vi "CONEX-CC Virtual Front Panel_v2.vi"(6 "+":bool, 7 "-":bool, 8 "Set velocity":bool, 9 "Action":bool) -> ()   [LabVIEW 2016]
doc: "CONEX - CC Virtual Front Panel:\n\nThis is a sample of an application that can be built with the LabVIEW drivers.\n\nPress HOME / ENABLE in top left of panel to put stage in Ready state for motion."
uses:
  <vilib>/Platform/TimedLoop/XDataNode/timing_clust.ctl
  <vilib>/Platform/TimedLoop/XDataNode/nitl_modes.ctl
  <vilib>/Platform/TimedLoop/XDataNode/wakeup.ctl
  <vilib>/Platform/TimedLoop/XDataNode/XDataNode.xnode
  <vilib>/Platform/TimedLoop/XDataNode/XDNodeRunTimeDep.lvlib
panel:
  out "Title":string
  out "counter":i32
  in  "Set Max":bool
  in  "Set Min":bool
  in  "Max":dbl
  in  "Min":dbl
  out "Stop cycle":bool=TRUE
  out "Title 2":string
  in  "Cycle":bool
  in  "# Loops":i32=5
  in  "Go2":bool
  in  "Go1":bool
  in  "Abs. Move 2":dbl=1.0
  in  "Abs. Move 1":dbl
  in  "Step":dbl
  out "Position History":dbl(graph)=1.5
  out "Stop polling":bool=TRUE
  out "Controller state description":string="STATUS"
  out "Velocity MAX":dbl=0.4
  out "Controller state":string="33"
  out "Positioner error":string="0000"
  in  "Velocity:":dbl
  in  "Exit":bool=TRUE
  out "Target position":dbl
  in  "Position glissière":cluster{dbl, dbl}(slide) scale=0.0..25.0
  in  "Exit":bool
  out "Current position":dbl
  # "unit/s"
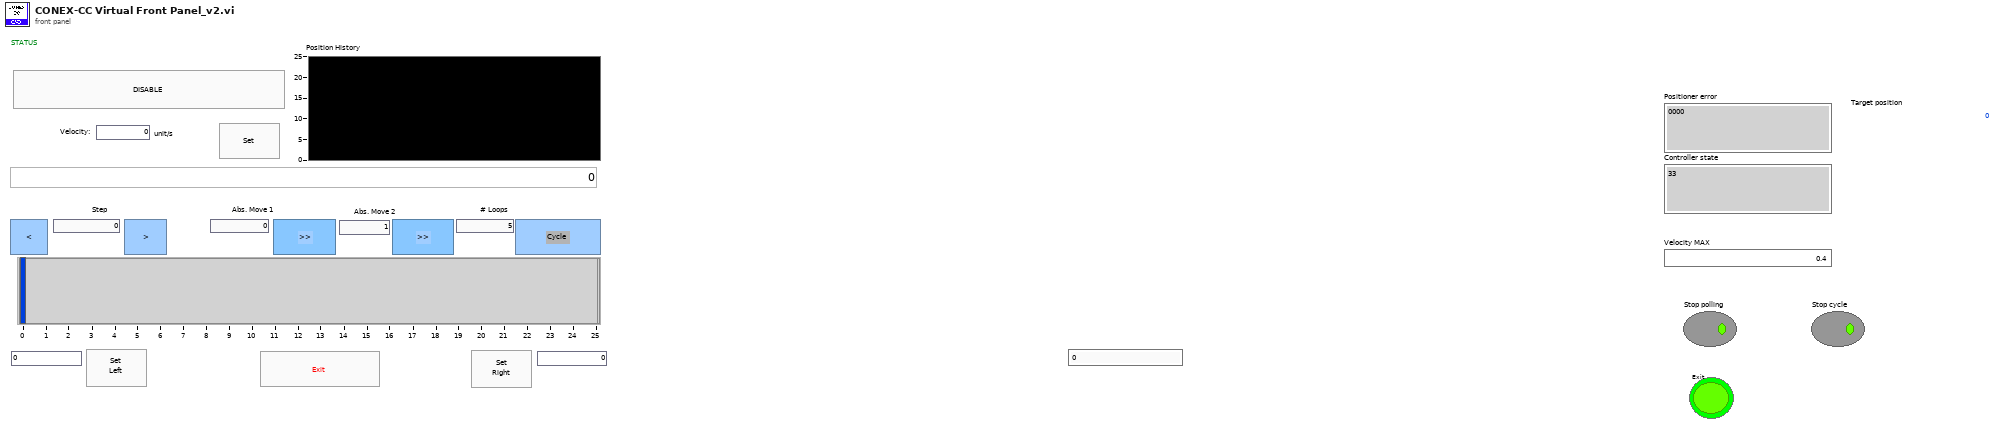
[diagram p1: front panel]
types:
  T1 = typedef "XDNodeRunTimeDep.lvlib/timing_clust.ctl" = cluster{"Expected End [f-1]":u64, "Actual End [f-1]":u64, "Finished Late? [f-1]":bool, "Expected End [i-1]":u64, "Actual End [i-1]":u64, "Finished Late? [i-1]":bool, "Expected Start [i]":u64, "Actual Start [i]":u64, "Expected Start [f]":u64, "Actual Start [f]":u64, "Source Name":string, "Structure Name":string, "Period":i64, "Deadline":i64, "Offset":i64, "Start":i64, "Priority":i32, "Timeout":i32, "Mode":T2, "Wakeup Reason":T3, "Error":errorcluster, "Source Type":string, "Secondary Source Type":string, "Global End Time":u64, "Global Start Time":u64, "Frame Duration":u64, "Iteration Duration":u64, "Assigned CPU":i32, "I/O Scan Engine Mode":u32}
  T2 = typedef "XDNodeRunTimeDep.lvlib/nitl_modes.ctl" = enum32{"No Change", "Process missed periods, maintain original phase", "Discard missed periods, maintain original phase", "Process missed periods, ignore original phase", "Discard missed periods, ignore original phase"}
  T3 = typedef "XDNodeRunTimeDep.lvlib/wakeup.ctl" = enum32{"Normal", "Aborted", "Asynchronous wakeup", "Timing source error", "Timed loop error", "Timeout"}
  T4 = cluster{"VISA resource name":refnum<visa-resource-name>, "Device name":string, "Controller address":i32, "error":errorcluster}
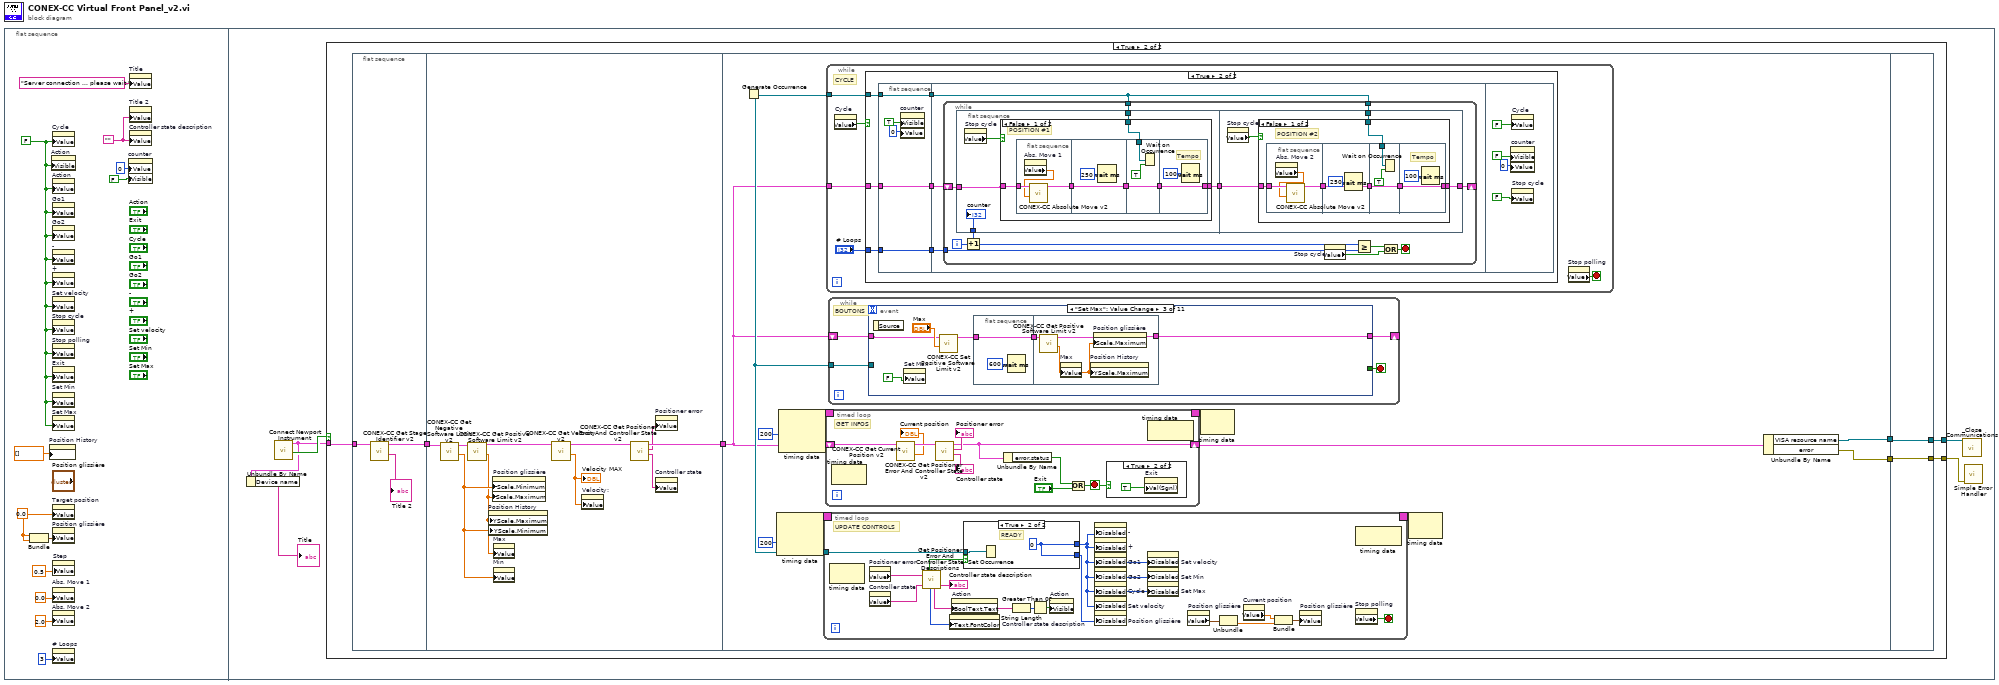
[diagram p0: block diagram]
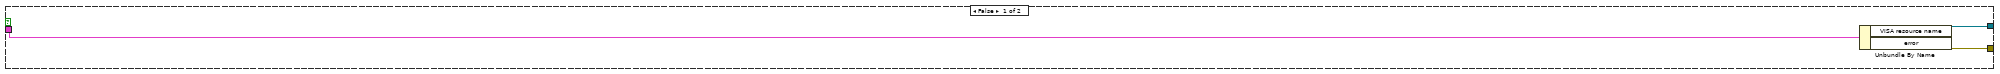
[diagram p2: hidden frame]
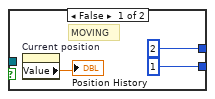
[diagram p6: hidden frame]
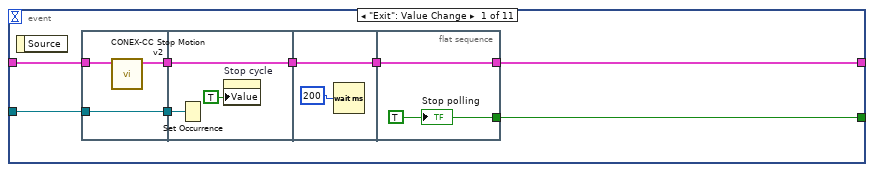
[diagram p7: hidden frame]
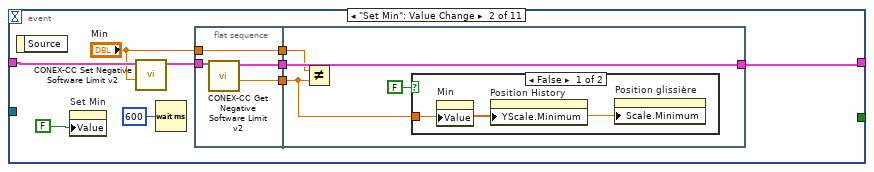
[diagram p8: hidden frame]
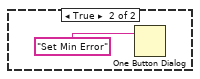
[diagram p9: hidden frame]
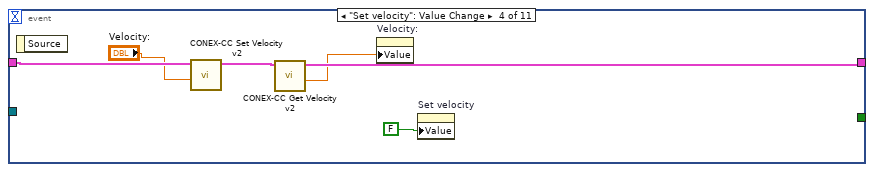
[diagram p10: hidden frame]
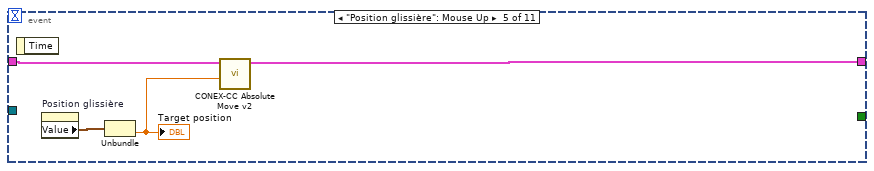
[diagram p11: hidden frame]
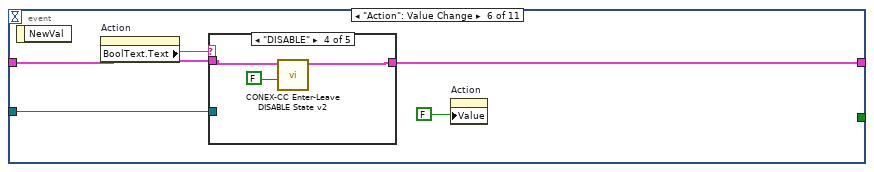
[diagram p12: hidden frame]
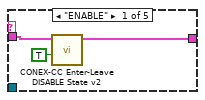
[diagram p13: hidden frame]
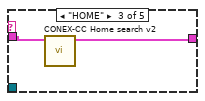
[diagram p15: hidden frame]
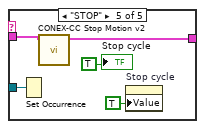
[diagram p16: hidden frame]
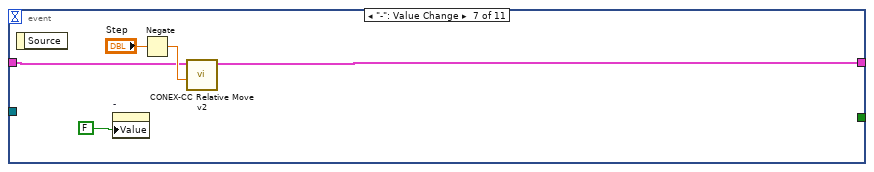
[diagram p17: hidden frame]
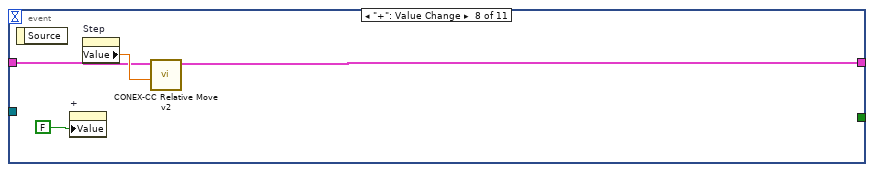
[diagram p18: hidden frame]
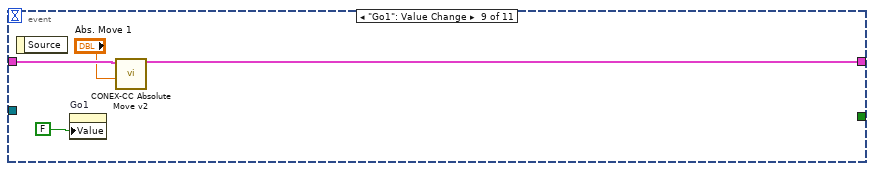
[diagram p19: hidden frame]
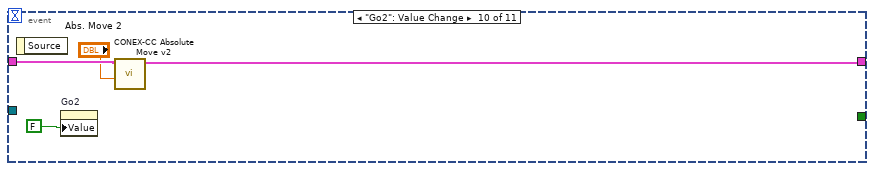
[diagram p20: hidden frame]
diagram:
  n1 = flat-sequence {
    frame #0 {
      w8 = FALSE
      w11 = 0.0
      w10 = ""
      n2 = Bundle(w11, w11) -> (w12:cluster{dbl, dbl})  [unwired: 1 out]
      n3 = property on="Position History" class="WFChart (strict)"("History Data"=dbl[] [] ("Données d'historique")) -> ()  [unwired: 2 in, 2 out]
      n4 = property on="Action" class="Bool (strict)"("Visible"=w8) -> ()  [unwired: 2 in, 2 out]
      n5 = property on="Cycle" class="Bool (strict)"("Value"=w8) -> ()  [unwired: 2 in, 2 out]
      n6 = property on="Action" class="Bool (strict)"("Value"=w8) -> ()  [unwired: 2 in, 2 out]
      n7 = property on="Go1" class="Bool (strict)"("Value"=w8) -> ()  [unwired: 2 in, 2 out]
      n8 = property on="Go2" class="Bool (strict)"("Value"=w8) -> ()  [unwired: 2 in, 2 out]
      n9 = property on="-" class="Bool (strict)"("Value"=w8) -> ()  [unwired: 2 in, 2 out]
      n10 = property on="+" class="Bool (strict)"("Value"=w8) -> ()  [unwired: 2 in, 2 out]
      n11 = property on="Set velocity" class="Bool (strict)"("Value"=w8) -> ()  [unwired: 2 in, 2 out]
      n12 = property on="Stop cycle" class="Bool (strict)"("Value"=w8) -> ()  [unwired: 2 in, 2 out]
      n13 = property on="Stop polling" class="Bool (strict)"("Value"=w8) -> ()  [unwired: 2 in, 2 out]
      n14 = property on="Exit" class="Bool (strict)"("Value"=w8) -> ()  [unwired: 2 in, 2 out]
      n15 = property on="Set Min" class="Bool (strict)"("Value"=w8) -> ()  [unwired: 2 in, 2 out]
      n16 = property on="Set Max" class="Bool (strict)"("Value"=w8) -> ()  [unwired: 2 in, 2 out]
      n17 = property on="Target position" class="DigNum (strict)"("Value"=w11) -> ()  [unwired: 2 in, 2 out]
      n18 = property on="Position glissière" class="Slide (strict)"("Value"=w12) -> ()  [unwired: 2 in, 2 out]
      n19 = property on="Abs. Move 1" class="DigNum (strict)"("Value"=0.0 ("Abs. Move 1")) -> ()  [unwired: 2 in, 2 out]
      n20 = property on="Abs. Move 2" class="DigNum (strict)"("Value"=2.0 ("Abs. Move 2")) -> ()  [unwired: 2 in, 2 out]
      n21 = property on="# Loops" class="DigNum (strict)"("Value"=3 ("# Loops")) -> ()  [unwired: 2 in, 2 out]
      n22 = property on="Step" class="DigNum (strict)"("Value"=0.5 ("Step")) -> ()  [unwired: 2 in, 2 out]
      n23 = property on="counter" class="DigNum (strict)"("Value"=0 ("counter"), "Visible"=FALSE) -> ()  [unwired: 2 in, 2 out]
      n24 = property on="Title" class="Str"("Value"="Server connection ... please wait." ("Title")) -> ()  [unwired: 2 in, 2 out]
      n25 = property on="Title 2" class="Str"("Value"=w10) -> ()  [unwired: 2 in, 2 out]
      n26 = property on="Controller state description" class="Str"("Value"=w10) -> ()  [unwired: 2 in, 2 out]
    }
    frame #1 {
      n27 = call <userlib>:"Connect Newport Instrument.vi"() -> ("Connected"=w15:bool, "Device Connection Cluster"=w14:T4)  [unwired: 7 in, 3 out]
      n28 = Unbundle By Name(w14) -> ("Device name"=→"Title":string)
      n29 = case shown="True" w15 {
        tunnel: [w19 w27] -> w17
        tunnel: w14 -> [w20 w25]
        tunnel: [w18 w21] -> w13
        frame False {
          n30 = Unbundle By Name(w20) -> ("VISA resource name"=w18:refnum<visa-resource-name>, "error"=w19:errorcluster)
        }
        frame True {
          n31 = flat-sequence {
            tunnel: w25 -> [w30]
            tunnel: [w28] -> w24
            tunnel: [w37] -> w26
            tunnel: w24 -> [w34]
            tunnel: w26 -> [w41]
            tunnel: [w43] -> w23
            tunnel: [w42] -> w22
            tunnel: [w273] -> w27
            tunnel: w23 -> [w272]
            tunnel: w22 -> [w273]
            tunnel: [w272] -> w21
            frame #0 {
              n32 = call <userlib>:"CONEX-CC Get Stage Identifier v2.vi"("Connection Cluster in"=w30) -> ("Identifier"=→"Title 2":string, "Connection Cluster out"=w28:T4)  [unwired: 9 in]
            }
            frame #1 {
              n33 = call <userlib>:"CONEX-CC Get Negative Software Limit v2.vi"("Connection Cluster in"=w34) -> ("Left limit"=w39:dbl, "Connection Cluster out"=w33:T4)  [unwired: 9 in]
              n34 = call <userlib>:"CONEX-CC Get Positive Software Limit v2.vi"("Connection Cluster in"=w33) -> ("Right limit"=w38:dbl, "Connection Cluster out"=w32:T4)  [unwired: 9 in]
              n35 = property on="Position History" class="WFChart (strict)"("YScale.Maximum"=w38, "YScale.Minimum"=w39) -> ()  [unwired: 2 in, 2 out]
              n36 = property on="Position glissière" class="Slide (strict)"("Scale.Minimum"=w39, "Scale.Maximum"=w38) -> ()  [unwired: 2 in, 2 out]
              n37 = property on="Max" class="DigNum (strict)"("Value"=w38) -> ()  [unwired: 2 in, 2 out]
              n38 = property on="Min" class="DigNum (strict)"("Value"=w39) -> ()  [unwired: 2 in, 2 out]
              n39 = call <userlib>:"CONEX-CC Get Velocity v2.vi"("Connection Cluster in"=w32) -> ("Velocity"=w40:dbl, "Connection Cluster out"=w31:T4)  [unwired: 8 in, 1 out]
              "Velocity MAX" <- w40
              n40 = property on="Velocity:" class="DigNum (strict)"("Value"=w40) -> ()  [unwired: 2 in, 2 out]
              n41 = call <userlib>:"CONEX-CC Get Positioner Error And Controller State v2.vi"("Connection Cluster in"=w31) -> ("Controller state"=w35:string, "Positioner error"=w36:string, "Connection Cluster out"=w37:T4)  [unwired: 8 in]
              n42 = property on="Positioner error" class="Str"("Value"=w36) -> ()  [unwired: 2 in, 2 out]
              n43 = property on="Controller state" class="Str"("Value"=w35) -> ()  [unwired: 2 in, 2 out]
            }
            frame #2 {
              n44 = Generate Occurrence() -> (w45:refnum<k4>)
              n45 = node-c288(i64 200 ("Période")) -> (w49:T1)  [unwired: 1 in, 1 out]
              n46 = node-c288(i64 200 ("Période")) -> (w51:T1)  [unwired: 1 in, 1 out]
              n47 = timed-loop {
                timing: w49 -> [_]
                timing-out: [_] -> w48
                tunnel: w45 -> [w133]
                stop <- w135 stop-if-true
                # "UPDATE CONTROLS"
                n48 = node-c288() -> ()  [unwired: 2 out]
                n49 = property on="Positioner error" class="Str"() -> ("Value"=w144:string)  [unwired: 2 in, 2 out]
                n50 = property on="Controller state" class="Str"() -> ("Value"=w143:string)  [unwired: 2 in, 2 out]
                n51 = call <userlib>:"Get Positioner Error And Controller State Descriptions.vi"("Controller state"=w143, "Positioner error"=w144) -> ("Color"=w141:u32, "Action name"=w140:string, "Controller state description"=→"Controller state description":string, "IsReady?"=w137:bool)  [unwired: 2 out]
                n52 = property on="Controller state description" class="Str"("Text.FontColor"=w141) -> ()  [unwired: 2 in, 2 out]
                n53 = property on="Action" class="Bool (strict)"("BoolText.Text"=w140) -> ()  [unwired: 2 in, 2 out]
                n54 = case shown="True" w137 {
                  tunnel: [u8 2 w149] -> w134
                  tunnel: [u8 1 w149] -> w136
                  tunnel: w133 -> [_ w148]
                  frame False {
                    # "MOVING"
                    n55 = property on="Current position" class="DigNum (strict)"() -> ("Value"=→"Position History":dbl)  [unwired: 2 in, 2 out]
                  }
                  frame True {
                    w149 = u8 0
                    # "READY"
                    n56 = Set Occurrence(w148) -> ()
                  }
                }
                n57 = String Length(string=w140) -> (length=w139:i32)
                n58 = Greater Than 0?(x=w139) -> (x > 0?=w138:bool)
                n59 = property on="Action" class="Bool (strict)"("Visible"=w138) -> ()  [unwired: 2 in, 2 out]
                n60 = property on="-" class="Bool (strict)"("Disabled"=w134) -> ()  [unwired: 2 in, 2 out]
                n61 = property on="+" class="Bool (strict)"("Disabled"=w134) -> ()  [unwired: 2 in, 2 out]
                n62 = property on="Go1" class="Bool (strict)"("Disabled"=w134) -> ()  [unwired: 2 in, 2 out]
                n63 = property on="Go2" class="Bool (strict)"("Disabled"=w134) -> ()  [unwired: 2 in, 2 out]
                n64 = property on="Cycle" class="Bool (strict)"("Disabled"=w134) -> ()  [unwired: 2 in, 2 out]
                n65 = property on="Set velocity" class="Bool (strict)"("Disabled"=w134) -> ()  [unwired: 2 in, 2 out]
                n66 = property on="Position glissière" class="Slide (strict)"("Disabled"=w136) -> ()  [unwired: 2 in, 2 out]
                n67 = property on="Set velocity" class="Bool (strict)"("Disabled"=w134) -> ()  [unwired: 2 in, 2 out]
                n68 = property on="Set Min" class="Bool (strict)"("Disabled"=w134) -> ()  [unwired: 2 in, 2 out]
                n69 = property on="Set Max" class="Bool (strict)"("Disabled"=w134) -> ()  [unwired: 2 in, 2 out]
                n70 = property on="Position glissière" class="Slide (strict)"() -> ("Value"=w130:cluster{dbl, dbl})  [unwired: 2 in, 2 out]
                n71 = Unbundle(w130) -> (w129:dbl)  [unwired: 1 out]
                n72 = property on="Current position" class="DigNum (strict)"() -> ("Value"=w131:dbl)  [unwired: 2 in, 2 out]
                n73 = Bundle("Value"=w131, w129) -> (w132:cluster{"Value":dbl, dbl})  [unwired: 1 out]
                n74 = property on="Position glissière" class="Slide (strict)"("Value"=w132) -> ()  [unwired: 2 in, 2 out]
                n75 = node-c288() -> ()  [unwired: 2 out]
                n76 = property on="Stop polling" class="Bool (strict)"() -> ("Value"=w135:bool)  [unwired: 2 in, 2 out]
              }
              n77 = timed-loop {
                timing: w51 -> [_]
                timing-out: [_] -> w50
                shift-right: [w258] -> w44
                shift-left: w41 -> [w260]
                stop <- w262 stop-if-true
                # "GET INFOS"
                n78 = node-c288() -> ()  [unwired: 2 out]
                n79 = call <userlib>:"CONEX-CC Get Current Position v2.vi"("Connection Cluster in"=w260) -> ("Current position"=→"Current position":dbl, "Connection Cluster out"=w259:T4)  [unwired: 8 in, 1 out]
                n80 = call <userlib>:"CONEX-CC Get Positioner Error And Controller State v2.vi"("Connection Cluster in"=w259) -> ("Controller state"=→"Controller state":string, "Positioner error"=→"Positioner error":string, "Connection Cluster out"=w258:T4)  [unwired: 8 in]
                n81 = Unbundle By Name(w258) -> ("error.status"=w257:bool)
                n82 = Or(x=w257, y="Exit") -> (x .or. y?=w262:bool)
                n83 = case shown="True" w262 {
                  frame False {
                  }
                  frame True {
                    n84 = property on="Exit" class="Bool (strict)"("Val(Sgnl)"=TRUE) -> ()  [unwired: 2 in, 2 out]
                  }
                }
                n85 = node-c288() -> ()  [unwired: 2 out]
              }
              n86 = while {
                tunnel: w41 -> [w56]
                tunnel: w45 -> [w52]
                stop <- w55 stop-if-true
                # "CYCLE"
                n87 = property on="Cycle" class="Bool (strict)"() -> ("Value"=w54:bool)  [unwired: 2 in, 2 out]
                n88 = case shown="True" w54 {
                  tunnel: w56 -> [_ w62]
                  tunnel: "# Loops" -> [_ w61]
                  tunnel: w52 -> [_ w58]
                  frame False {
                  }
                  frame True {
                    n89 = flat-sequence {
                      tunnel: w61 -> [w66]
                      tunnel: w62 -> [w67]
                      tunnel: [w67] -> w60
                      tunnel: [w66] -> w59
                      tunnel: w58 -> [w63]
                      tunnel: [w63] -> w57
                      tunnel: w60 -> [w68]
                      tunnel: w59 -> [w70]
                      tunnel: w57 -> [w69]
                      frame #0 {
                        n90 = property on="counter" class="DigNum (strict)"("Visible"=TRUE, "Value"=0 ("counter")) -> ()  [unwired: 2 in, 2 out]
                      }
                      frame #1 {
                        n91 = while {
                          tunnel: w70 -> [w81]
                          shift-right: [w71] -> _
                          shift-left: w68 -> [w72]
                          tunnel: w69 -> [w77]
                          tunnel: w69 -> [w76]
                          i -> [w75]
                          stop <- w80 stop-if-true
                          n92 = flat-sequence {
                            tunnel: [w86] -> w73
                            tunnel: w77 -> [w84]
                            tunnel: w74 -> [w83]
                            tunnel: w72 -> [w82]
                            tunnel: w73 -> [w107]
                            tunnel: w76 -> [w105]
                            tunnel: [w104] -> w71
                            frame #0 {
                              n93 = property on="Stop cycle" class="Bool (strict)"() -> ("Value"=w85:bool)  [unwired: 2 in, 2 out]
                              n94 = case shown="False" w85 {
                                tunnel: w82 -> [w92 w103]
                                tunnel: [w91 w103] -> w86
                                tunnel: w84 -> [w90 _]
                                frame False {
                                # "POSITION #1"
                                n95 = flat-sequence {
                                tunnel: w92 -> [w94]
                                tunnel: [w95] -> w89
                                tunnel: w89 -> [w97]
                                tunnel: [w97] -> w88
                                tunnel: w88 -> [w100]
                                tunnel: w90 -> [w98]
                                tunnel: [w100] -> w87
                                tunnel: [w102] -> w91
                                tunnel: w87 -> [w102]
                                frame #0 {
                                n96 = property on="Abs. Move 1" class="DigNum (strict)"() -> ("Value"=w93:dbl)  [unwired: 2 in, 2 out]
                                n97 = call <userlib>:"CONEX-CC Absolute Move v2.vi"("Target position"=w93, "Connection Cluster in"=w94) -> ("Connection Cluster out"=w95:T4)  [unwired: 5 in, 2 out]
                                }
                                frame #1 {
                                n98 = Wait (ms)(milliseconds to wait=u32 250 ("attente (ms)")) -> ()  [unwired: 1 out]
                                }
                                frame #2 {
                                n99 = Wait on Occurrence(1:TRUE ("ignorer les précédents (V)"), 2:w98) -> ()  [unwired: 1 in, 1 out]
                                }
                                frame #3 {
                                # "Tempo"
                                n100 = Wait (ms)(milliseconds to wait=u32 100 ("attente (ms)")) -> ()  [unwired: 1 out]
                                }
                                }
                                }
                                frame True {
                                }
                              }
                              "counter" <- w83
                            }
                            frame #1 {
                              n101 = property on="Stop cycle" class="Bool (strict)"() -> ("Value"=w106:bool)  [unwired: 2 in, 2 out]
                              n102 = case shown="False" w106 {
                                tunnel: w107 -> [w113 w124]
                                tunnel: w105 -> [w112 _]
                                tunnel: [w111 w124] -> w104
                                frame False {
                                # "POSITION #2"
                                n103 = flat-sequence {
                                tunnel: w113 -> [w116]
                                tunnel: [w115] -> w108
                                tunnel: [w117] -> w109
                                tunnel: w108 -> [w117]
                                tunnel: w112 -> [w121]
                                tunnel: [w119] -> w110
                                tunnel: w109 -> [w119]
                                tunnel: [w122] -> w111
                                tunnel: w110 -> [w122]
                                frame #0 {
                                n104 = property on="Abs. Move 2" class="DigNum (strict)"() -> ("Value"=w114:dbl)  [unwired: 2 in, 2 out]
                                n105 = call <userlib>:"CONEX-CC Absolute Move v2.vi"("Target position"=w114, "Connection Cluster in"=w116) -> ("Connection Cluster out"=w115:T4)  [unwired: 5 in, 2 out]
                                }
                                frame #1 {
                                n106 = Wait (ms)(milliseconds to wait=u32 250 ("attente (ms)")) -> ()  [unwired: 1 out]
                                }
                                frame #2 {
                                n107 = Wait on Occurrence(1:TRUE ("ignorer les précédents (V)"), 2:w121) -> ()  [unwired: 1 in, 1 out]
                                }
                                frame #3 {
                                # "Tempo"
                                n108 = Wait (ms)(milliseconds to wait=u32 100 ("attente (ms)")) -> ()  [unwired: 1 out]
                                }
                                }
                                }
                                frame True {
                                }
                              }
                            }
                          }
                          n109 = Increment(x=w75) -> (x+1=w74:i32)
                          n110 = property on="Stop cycle" class="Bool (strict)"() -> ("Value"=w78:bool)  [unwired: 2 in, 2 out]
                          n111 = Greater Or Equal?(x=w74, y=w81) -> (x >= y?=w79:bool)
                          n112 = Or(x=w79, y=w78) -> (x .or. y?=w80:bool)
                        }
                      }
                      frame #2 {
                        n113 = property on="counter" class="DigNum (strict)"("Visible"=FALSE, "Value"=0 ("counter")) -> ()  [unwired: 2 in, 2 out]
                        n114 = property on="Cycle" class="Bool (strict)"("Value"=FALSE ("Cycle")) -> ()  [unwired: 2 in, 2 out]
                        n115 = property on="Stop cycle" class="Bool (strict)"("Value"=FALSE ("Cycle")) -> ()  [unwired: 2 in, 2 out]
                      }
                    }
                  }
                }
                n116 = property on="Stop polling" class="Bool (strict)"() -> ("Value"=w55:bool)  [unwired: 2 in, 2 out]
              }
              n117 = while {
                shift-right: [w159] -> _
                shift-left: w41 -> [w158]
                tunnel: w45 -> [w156]
                stop <- w157 stop-if-true
                # "BOUTONS"
                n118 = event shown="[2] \"Set Max\": Value Change" {
                  selector: _ -> [_ _ _ _ _ _ _ _ _ _ _]
                  dyn-events: _ -> [_ _ _ _ _ _ _ _ _ _ _]
                  timeout: _ -> [_ _ _ _ _ _ _ _ _ _ _]
                  tunnel: [w165 _ _ _ _ _ _ _ _ _ _] -> w157
                  tunnel: w158 -> [w160 w184 w198 w210 w216 w221 w237 w243 w248 w252 w254]
                  tunnel: [w167 w183 w197 w213 w215 w220 w241 w242 w246 w251 w254] -> w159
                  tunnel: w156 -> [w162 _ _ _ _ w218 _ _ _ _ _]
                  event "Exit": Value Change {
                    n119 = event-data() -> ()  [unwired: 2 out]
                    n120 = flat-sequence {
                      tunnel: [w170] -> w166
                      tunnel: w162 -> [w169]
                      tunnel: [w169] -> w161
                      tunnel: w160 -> [w168]
                      tunnel: w166 -> [w173]
                      tunnel: [w173] -> w164
                      tunnel: w161 -> [w171]
                      tunnel: w164 -> [w175]
                      tunnel: [w175] -> w163
                      tunnel: [w177] -> w167
                      tunnel: w163 -> [w177]
                      tunnel: [w176] -> w165
                      frame #0 {
                        n121 = call <userlib>:"CONEX-CC Stop Motion v2.vi"("Connection Cluster in"=w168) -> ("Connection Cluster out"=w170:T4)  [unwired: 10 in]
                      }
                      frame #1 {
                        n122 = Set Occurrence(w171) -> ()
                        n123 = property on="Stop cycle" class="Bool (strict)"("Value"=TRUE) -> ()  [unwired: 2 in, 2 out]
                      }
                      frame #2 {
                        n124 = Wait (ms)(milliseconds to wait=u32 200 ("attente (ms)")) -> ()  [unwired: 1 out]
                      }
                      frame #3 {
                        w176 = TRUE
                        "Stop polling" <- w176
                      }
                    }
                  }
                  event "Set Min": Value Change {
                    n125 = event-data() -> ()  [unwired: 2 out]
                    n126 = property on="Set Min" class="Bool (strict)"("Value"=FALSE ("Set Min")) -> ()  [unwired: 2 in, 2 out]
                    n127 = call <userlib>:"CONEX-CC Set Negative Software Limit v2.vi"("Negative limit (left)"="Min", "Connection Cluster in"=w184) -> ("Connection Cluster out"=w186:T4)  [unwired: 9 in]
                    n128 = Wait (ms)(milliseconds to wait=u32 600 ("attente (ms)")) -> ()  [unwired: 1 out]
                    n129 = flat-sequence {
                      tunnel: w186 -> [w190]
                      tunnel: [w189] -> w181
                      tunnel: [w188] -> w180
                      tunnel: "Min" -> [w188]
                      tunnel: [w187] -> w178
                      tunnel: [w194] -> w183
                      tunnel: w181 -> [w194]
                      tunnel: w180 -> [w193]
                      tunnel: w178 -> [w191]
                      frame #0 {
                        n130 = call <userlib>:"CONEX-CC Get Negative Software Limit v2.vi"("Connection Cluster in"=w190) -> ("Left limit"=w187:dbl, "Connection Cluster out"=w189:T4)  [unwired: 9 in]
                      }
                      frame #1 {
                        n131 = Not Equal?(x=w193, y=w191) -> ()  [unwired: 1 out]
                        n132 = case shown="False" FALSE {
                          tunnel: w191 -> [w195 _]
                          frame False {
                            n133 = property on="Min" class="DigNum (strict)"("Value"=w195) -> ()  [unwired: 2 in, 2 out]
                            n134 = property on="Position History" class="WFChart (strict)"("YScale.Minimum"=w195) -> ()  [unwired: 2 in, 2 out]
                            n135 = property on="Position glissière" class="Slide (strict)"("Scale.Minimum"=w195) -> ()  [unwired: 2 in, 2 out]
                          }
                          frame True {
                            n136 = One Button Dialog(message="Set Min Error") -> ()  [unwired: 1 in, 1 out]
                          }
                        }
                      }
                    }
                  }
                  event "Set Max": Value Change {
                    n137 = event-data() -> ()  [unwired: 2 out]
                    n138 = property on="Set Max" class="Bool (strict)"("Value"=FALSE ("Set Max")) -> ()  [unwired: 2 in, 2 out]
                    n139 = call <userlib>:"CONEX-CC Set Positive Software Limit v2.vi"("Positive limit (right)"="Max", "Connection Cluster in"=w198) -> ("Connection Cluster out"=w202:T4)  [unwired: 9 in]
                    n140 = flat-sequence {
                      tunnel: w202 -> [w204]
                      tunnel: [w204] -> w199
                      tunnel: [w207] -> w197
                      tunnel: w199 -> [w205]
                      frame #0 {
                        n141 = Wait (ms)(milliseconds to wait=u32 600 ("attente (ms)")) -> ()  [unwired: 1 out]
                      }
                      frame #1 {
                        n142 = call <userlib>:"CONEX-CC Get Positive Software Limit v2.vi"("Connection Cluster in"=w205) -> ("Right limit"=w206:dbl, "Connection Cluster out"=w207:T4)  [unwired: 9 in]
                        n143 = property on="Max" class="DigNum (strict)"("Value"=w206) -> ()  [unwired: 2 in, 2 out]
                        n144 = property on="Position History" class="WFChart (strict)"("YScale.Maximum"=w206) -> ()  [unwired: 2 in, 2 out]
                        n145 = property on="Position glissière" class="Slide (strict)"("Scale.Maximum"=w206) -> ()  [unwired: 2 in, 2 out]
                      }
                    }
                  }
                  event "Set velocity": Value Change {
                    n146 = event-data() -> ()  [unwired: 2 out]
                    n147 = call <userlib>:"CONEX-CC Set Velocity v2.vi"("Velocity"="Velocity:", "Connection Cluster in"=w210) -> ("Connection Cluster out"=w209:T4)  [unwired: 9 in]
                    n148 = call <userlib>:"CONEX-CC Get Velocity v2.vi"("Connection Cluster in"=w209) -> ("Velocity"=w212:dbl, "Connection Cluster out"=w213:T4)  [unwired: 8 in, 1 out]
                    n149 = property on="Velocity:" class="DigNum (strict)"("Value"=w212) -> ()  [unwired: 2 in, 2 out]
                    n150 = property on="Set velocity" class="Bool (strict)"("Value"=FALSE ("Set velocity")) -> ()  [unwired: 2 in, 2 out]
                  }
                  event "Position glissière": Mouse Up {
                    n151 = event-data() -> ()  [unwired: 2 out]
                    n152 = property on="Position glissière" class="Slide (strict)"() -> ("Value"=w217:cluster{dbl, dbl})  [unwired: 2 in, 2 out]
                    n153 = Unbundle(w217) -> (w214:dbl)  [unwired: 1 out]
                    "Target position" <- w214
                    n154 = call <userlib>:"CONEX-CC Absolute Move v2.vi"("Target position"=w214, "Connection Cluster in"=w216) -> ("Connection Cluster out"=w215:T4)  [unwired: 5 in, 2 out]
                  }
                  event "Action": Value Change {
                    n155 = event-data() -> ()  [unwired: 2 out]
                    n156 = property on="Action" class="Bool (strict)"() -> ("BoolText.Text"=w222:string)  [unwired: 2 in, 2 out]
                    n157 = case shown="\"DISABLE\"" w222 {
                      tunnel: w221 -> [w224 w226 w228 w231 w233]
                      tunnel: [w223 w226 w227 w230 w236] -> w220
                      tunnel: w218 -> [_ _ _ _ w234]
                      frame "ENABLE" {
                        n158 = call <userlib>:"CONEX-CC Enter-Leave DISABLE State v2.vi"("Ready? (false=DISABLE true=READY)"=TRUE ("Flag (false=DISABLE true=READY)"), "Connection Cluster in"=w224) -> ("Connection Cluster out"=w223:T4)  [unwired: 7 in]
                      }
                      frame Default {
                      }
                      frame "HOME" {
                        n159 = call <userlib>:"CONEX-CC Home search v2.vi"("Connection Cluster in"=w228) -> ("Connection Cluster out"=w227:T4)  [unwired: 5 in, 3 out]
                      }
                      frame "DISABLE" {
                        n160 = call <userlib>:"CONEX-CC Enter-Leave DISABLE State v2.vi"("Ready? (false=DISABLE true=READY)"=FALSE ("Flag (false=DISABLE true=READY)"), "Connection Cluster in"=w231) -> ("Connection Cluster out"=w230:T4)  [unwired: 7 in]
                      }
                      frame "STOP" {
                        n161 = Set Occurrence(w234) -> ()
                        n162 = call <userlib>:"CONEX-CC Stop Motion v2.vi"("Connection Cluster in"=w233) -> ("Connection Cluster out"=w236:T4)  [unwired: 10 in]
                        n163 = property on="Stop cycle" class="Bool (strict)"("Value"=TRUE) -> ()  [unwired: 2 in, 2 out]
                        "Stop cycle" <- TRUE ("Stop cycle")
                      }
                    }
                    n164 = property on="Action" class="Bool (strict)"("Value"=FALSE) -> ()  [unwired: 2 in, 2 out]
                  }
                  event "-": Value Change {
                    n165 = event-data() -> ()  [unwired: 2 out]
                    n166 = property on="-" class="Bool (strict)"("Value"=FALSE ("-")) -> ()  [unwired: 2 in, 2 out]
                    n167 = Negate(x="Step") -> (-x=w239:dbl)
                    n168 = call <userlib>:"CONEX-CC Relative Move v2.vi"("Relative displacement"=w239, "Connection Cluster in"=w237) -> ("Connection Cluster out"=w241:T4)  [unwired: 9 in]
                  }
                  event "+": Value Change {
                    n169 = event-data() -> ()  [unwired: 2 out]
                    n170 = property on="+" class="Bool (strict)"("Value"=FALSE ("+")) -> ()  [unwired: 2 in, 2 out]
                    n171 = property on="Step" class="DigNum (strict)"() -> ("Value"=w245:dbl)  [unwired: 2 in, 2 out]
                    n172 = call <userlib>:"CONEX-CC Relative Move v2.vi"("Relative displacement"=w245, "Connection Cluster in"=w243) -> ("Connection Cluster out"=w242:T4)  [unwired: 9 in]
                  }
                  event "Go1": Value Change {
                    n173 = event-data() -> ()  [unwired: 2 out]
                    n174 = property on="Go1" class="Bool (strict)"("Value"=FALSE ("Go1")) -> ()  [unwired: 2 in, 2 out]
                    n175 = call <userlib>:"CONEX-CC Absolute Move v2.vi"("Target position"="Abs. Move 1", "Connection Cluster in"=w248) -> ("Connection Cluster out"=w246:T4)  [unwired: 5 in, 2 out]
                  }
                  event "Go2": Value Change {
                    n176 = event-data() -> ()  [unwired: 2 out]
                    n177 = property on="Go2" class="Bool (strict)"("Value"=FALSE ("Go2")) -> ()  [unwired: 2 in, 2 out]
                    n178 = call <userlib>:"CONEX-CC Absolute Move v2.vi"("Target position"="Abs. Move 2", "Connection Cluster in"=w252) -> ("Connection Cluster out"=w251:T4)  [unwired: 5 in, 2 out]
                  }
                  event "Cycle": Value Change {
                    (unwired) 0 ("Numérique")
                    n179 = event-data() -> ()  [unwired: 2 out]
                    n180 = property on="Cycle" class="Bool (strict)"("Value"=TRUE ("Cycle")) -> ()  [unwired: 2 in, 2 out]
                  }
                }
              }
              n181 = node-c288(w50) -> ()  [unwired: 1 out]
              n182 = node-c288(w48) -> ()  [unwired: 1 out]
              n183 = Unbundle By Name(w44) -> ("VISA resource name"=w43:refnum<visa-resource-name>, "error"=w42:errorcluster)
            }
            frame #3 {
            }
          }
        }
      }
      n184 = call <userlib>:"_Close Communications.vi"("Instrument Channel"=w13) -> ()  [unwired: 14 in, 1 out]
      n185 = call <vilib>:"Simple Error Handler.vi"("error in (no error)"=w17) -> ()  [unwired: 1 in, 8 out]
    }
  }
